vi "Acquire data triggered.vi"() -> ()   [LabVIEW 2020]
uses:
  <vilib>/Utility/error.llb/DialogType.ctl
  <vilib>/DAQmx/read.llb/DAQmx Read (Analog 1D Wfm NChan NSamp).vi
  <vilib>/DAQmx/create/channels.llb/DAQmx Create Channel (AI-Voltage-Basic).vi
  <vilib>/DAQmx/configure/timing.llb/DAQmx Timing (Sample Clock).vi
  <vilib>/DAQmx/configure/task.llb/DAQmx Configure Logging (TDMS).vi
  <vilib>/DAQmx/configure/trigger.llb/DAQmx Start Trigger (Digital Edge).vi
  <vilib>/DAQmx/miscellaneous.llb/DAQmx Fill In Error Info.vi
  <resource>/objmgr/daqmx.rc
panel:
  in  "trigger source":tag
  in  "stop":bool
  out "Waveform Graph":waveform(dbl)[](graph)
  in  "Number of Samples":i32=100
  in  "TDMS File Path":path
  in  "Sample Rate":dbl=1000.0
  in  "Sample Clock Source":tag="OnboardClock"
  in  "Terminal Configuration":i32(ring)=-1 items=["default"=-1, "RSE"=10083, "NRSE"=10078, "Differential"=10106, "Pseudodifferential"=12529]
  in  "Max Voltage":dbl=5.0
  in  "Min Voltage":dbl=-5.0
  in  "Physical Channel":tag="Dev1/ai0"
  out "Actual Sample Rate":dbl=1000.0 format="%0.2f"
  in  "Logging Mode":i32(ring)=10231 items=["Off"=10231, "Log and Read"=15842]
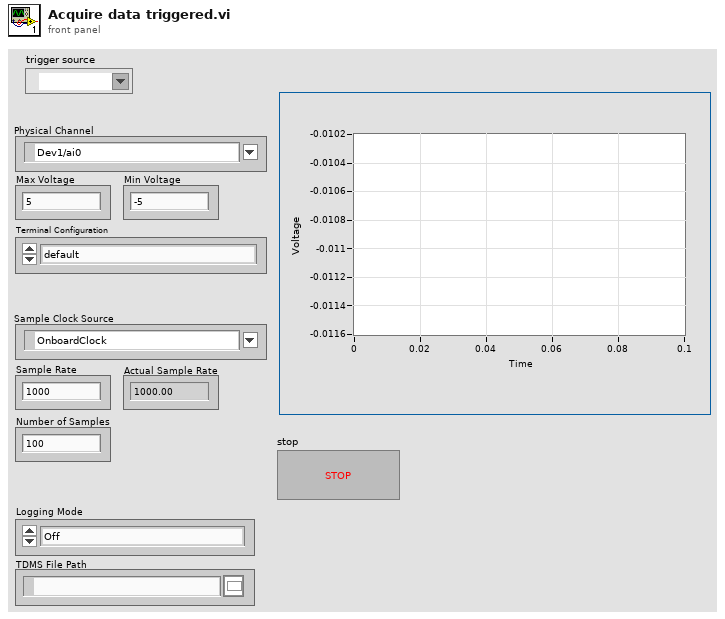
[diagram p1: front panel]
types:
  T1 = typedef "DialogType.ctl" = u16
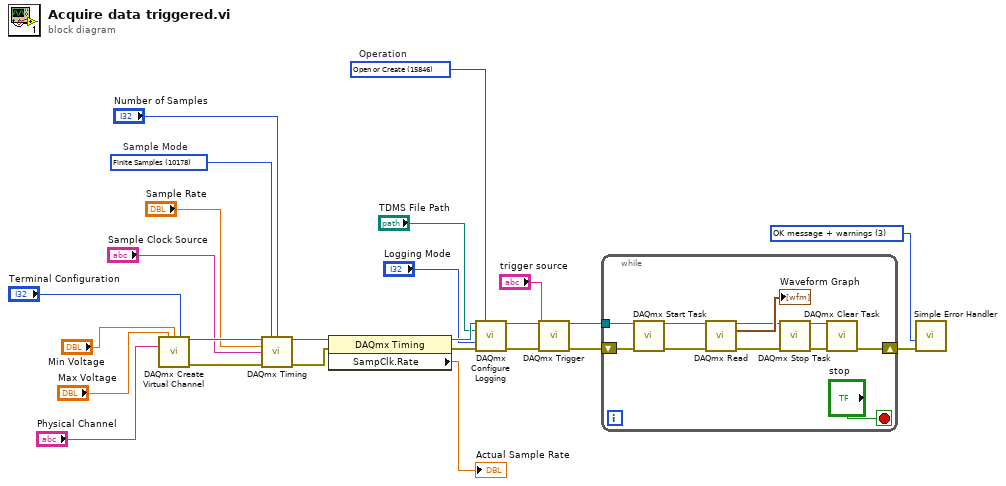
[diagram p0: block diagram]
diagram:
  w2 = T1 3 items=["no dialog", "OK message", "continue or stop message", "OK message + warnings", "continue/stop + warnings"] ("type of dialog (OK msg:1)")
  w18 = 15846 items=["Open"=10437, "Open or Create"=15846, "Create or Replace"=15847, "Create"=15848]  # Operation
  w23 = 10178 items=["Finite Samples"=10178, "Continuous Samples"=10123, "Hardware Timed Single Point"=12522]  # Sample Mode
  n1 = call-poly <vilib>:"DAQmx Create Virtual Channel.vi"("maximum value"="Max Voltage", "minimum value"="Min Voltage", "input terminal configuration"="Terminal Configuration", "physical channels"="Physical Channel") -> ("task out"=w21:refnum<k21>, "error out"=w22:errorcluster)  [unwired: 10 in]
  n2 = call-poly <vilib>:"DAQmx Timing.vi"("task/channels in"=w21, "sample mode"=w23, "samples per channel"="Number of Samples", "rate"="Sample Rate", "source"="Sample Clock Source", "error in"=w22) -> ("task out"=w25:refnum<k21>, "error out"=w24:errorcluster)  [unwired: 8 in]
  n3 = property class="DAQmx Timing"(reference=w25, error in=w24) -> (reference out=w20:refnum<k21>, error out=w19:errorcluster, "SampClk.Rate"=→"Actual Sample Rate":dbl)
  n4 = call-poly <vilib>:"DAQmx Configure Logging.vi"("task/channels in"=w20, "operation"=w18, "file path"="TDMS File Path", "logging mode"="Logging Mode", "error in"=w19) -> ("task out"=w6:refnum<k21>, "error out"=w5:errorcluster)  [unwired: 9 in]
  n5 = call-poly <vilib>:"DAQmx Trigger.vi"("task/channels in"=w6, "source"="trigger source", "error in"=w5) -> ("task out"=w4:refnum<k21>, "error out"=w3:errorcluster)  [unwired: 11 in]
  n6 = while {
    tunnel: w4 -> [w28]
    shift-right: [w34] -> w17
    shift-left: w3 -> [w27]
    stop <- "stop" stop-if-true
    n7 = call <vilib>:"DAQmx Start Task.vi"("task/channels in"=w28, "error in"=w27) -> ("task out"=w36:refnum<k21>, "error out"=w35:errorcluster)  [unwired: 12 in]
    n8 = call-poly <vilib>:"DAQmx Read.vi"("task/channels in"=w36, "error in"=w35) -> ("task out"=w30:refnum<k21>, "data"=→"Waveform Graph":waveform(dbl)[], "error out"=w29:errorcluster)  [unwired: 11 in]
    n9 = call <vilib>:"DAQmx Stop Task.vi"("task/channels in"=w30, "error in"=w29) -> ("task out"=w32:refnum<k21>, "error out"=w31:errorcluster)  [unwired: 12 in]
    n10 = call <vilib>:"DAQmx Clear Task.vi"("task in"=w32, "error in"=w31) -> ("error out"=w34:errorcluster)  [unwired: 13 in]
  }
  n11 = call <vilib>:"Simple Error Handler.vi"("type of dialog (OK msg:1)"=w2, "error in (no error)"=w17) -> ()  [unwired: 3 in, 5 out]
